vi "step5 AlignFrontEdge.vi"(8 "error in (no error)":errorcluster, 11 "cube in":T1) -> (0 "error out":errorcluster, 3 "cube out":T1)   [LabVIEW 2011]
doc: "Rotate cube as necessary so that the top middle piece matches the desired start colour.\n\nNo transformations are done in this VI, the operations are loaded on the the operation queue bus."
uses:
  Typedef/cube.ctl
  Typedef/face.ctl
  Typedef/operation.ctl
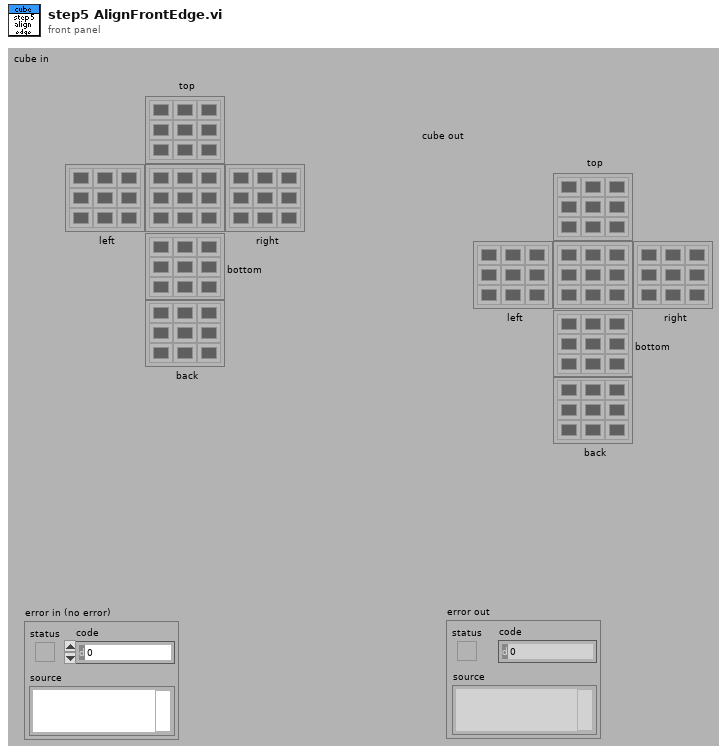
[diagram p1: front panel]
types:
  T1 = typedef "cube.ctl" = cluster{"top":T2, "left":T2, "right":T2, "bottom":T2, "back":T2, "front":T2}
  T2 = typedef "face.ctl" = u32[][]
  T3 = typedef "operation.ctl" = enum16{"nop", "T+", "T-", "F+", "F-", "L+", "L-", "R+", "R-", "B+", "B-", "<--", "-->", "^", "V"}
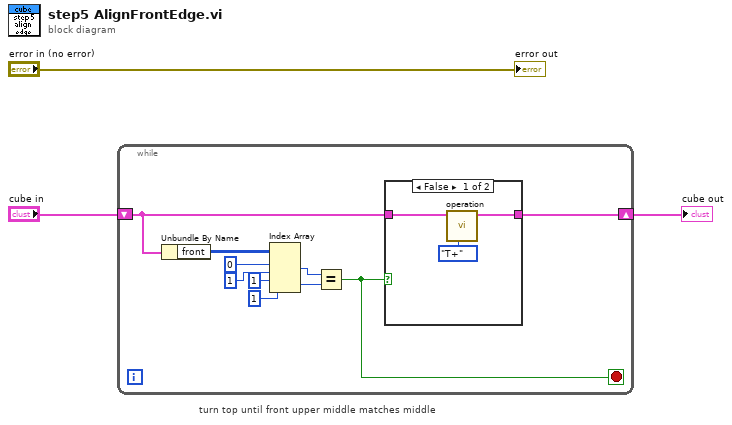
[diagram p0: block diagram]
diagram:
  # "turn top until front upper middle matches middle"
  n1 = while {
    shift-right: [w7] -> w1
    shift-left: "cube in" -> [w5]
    stop <- w6 stop-if-true
    n2 = Unbundle By Name(w5) -> ("front"=w4:T2)
    n3 = Index Array(array=w4, index (row) #1=0 ("index (row)"), index (col) #1=1 ("disabled index (col)"), index (row) #2=1 ("index (row)"), index (col) #2=1 ("disabled index (col)")) -> (element #1=w12:u32, element #2=w13:u32)
    n4 = Equal?(x=w12, y=w13) -> (x = y?=w6:bool)
    n5 = case shown="False" w6 {
      tunnel: w5 -> [w15 w17]
      tunnel: [w14 w17] -> w7
      frame False {
        n6 = call "operation.vi"("operation"=operation."T+", "cube in"=w15) -> ("cube out"=w14:T1)  [unwired: 8 in, 1 out]
      }
      frame True {
      }
    }
  }
  "cube out" <- w1
  "error out" <- "error in (no error)"
